vi "load_top_level_configuration.vi"(7 "force load?":bool=TRUE, 8 "error in (no error)":errorcluster, 11 "user":string) -> (0 "error out":errorcluster, 3 "configuration":T1)   [LabVIEW 2010]
uses:
  type_definitions/clusters/top_level_config_cluster.ctl
  common/clusters/plugin_specification.ctl
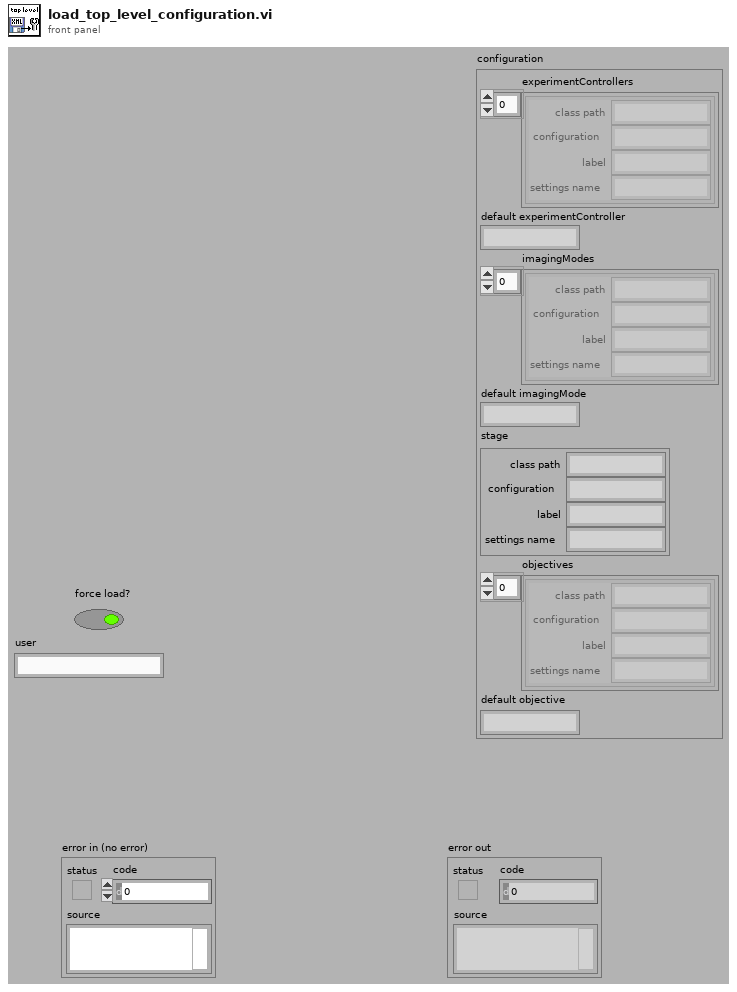
[diagram p1: front panel]
types:
  T1 = typedef "top_level_config_cluster.ctl" = cluster{"experimentControllers":T2[], "default experimentController":string, "imagingModes":T2[], "default imagingMode":string, "stage":T2, "objectives":T2[], "default objective":string}
  T2 = typedef "plugin_specification.ctl" = cluster{"class path":string, "configuration":string, "label":string, "settings name":string}
  T3 = typedef "configuration_paths_cluster.ctl" = cluster{"base folder":path, "base folder for user":path, "component folder":path, "component file path":path, "main folder":path, "main file":path}
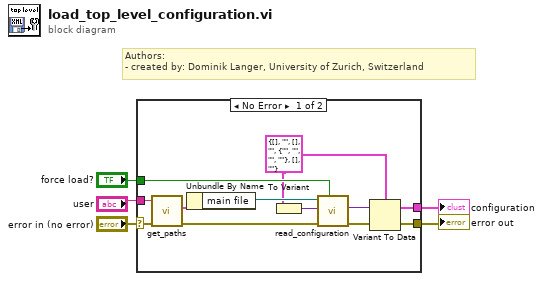
[diagram p0: block diagram]
diagram:
  # "Authors: \n- created by: Dominik Langer, University of Zurich, Switzerland"
  n1 = case shown="No Error" "error in (no error)" {
    selector: "error in (no error)" -> [w17 w18]
    tunnel: [w7 w18] -> w4
    tunnel: [w9 _] -> w3
    tunnel: "force load?" -> [w13 _]
    tunnel: "user" -> [w6 _]
    frame No Error {
      w10 = T1 {"experimentControllers"=[], "default experimentController"="", "imagingModes"=[], "default imagingMode"="", "stage"={"class path"="", "configuration"="", "label"="", "settings name"=""}, "objectives"=[], "default objective"=""} ("configuration")
      n2 = call "get_paths.vi"("error in (no error)"=w17, "user"=w6) -> ("error out"=w16:errorcluster, "configuration paths"=w15:T3)  [unwired: 6 in, 2 out]
      n3 = Unbundle By Name(w15) -> ("main file"=w14:path)
      n4 = To Variant(anything=w10) -> (Variant=w12:variant)
      n5 = call "read_configuration.vi"("force load?"=w13, "error in (no error)"=w16, "config cluster variant in (data type)"=w12, "path"=w14) -> ("error out"=w8:errorcluster, "config cluster variant out (populated"=w11:variant)  [unwired: 3 in, 3 out]
      n6 = Variant To Data(error in=w8, Variant=w11, type=w10) -> (error out=w7:errorcluster, data=w9:T1)
    }
    frame Error {
    }
  }
  "error out" <- w4
  "configuration" <- w3
